vi "SeqMgr.Variables - Add, Replace.vi"(8 "error in (no error)":errorcluster, 9 "Name, Value":string[][](array[string]), 10 "Init":bool, 11 "SeqMgr in":refnum<class "SeqMgr.lvclass">) -> (0 "error out":errorcluster, 3 "SeqMgr out":refnum<class "SeqMgr.lvclass">)   [LabVIEW 2024, in "EQMF.lvlib" / "SeqMgr.lvlib" / "SeqMgr.lvclass"]
uses:
  SeqMgr.lvclass
  SeqMgr.lvclass/SeqMgr.ctl
  Strings/String Utils.lvlib
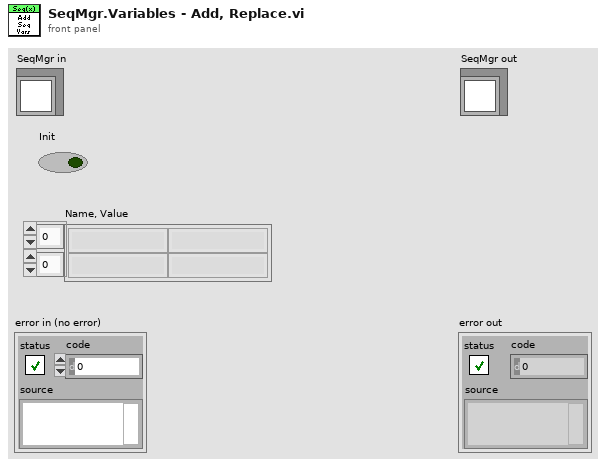
[diagram p1: front panel]
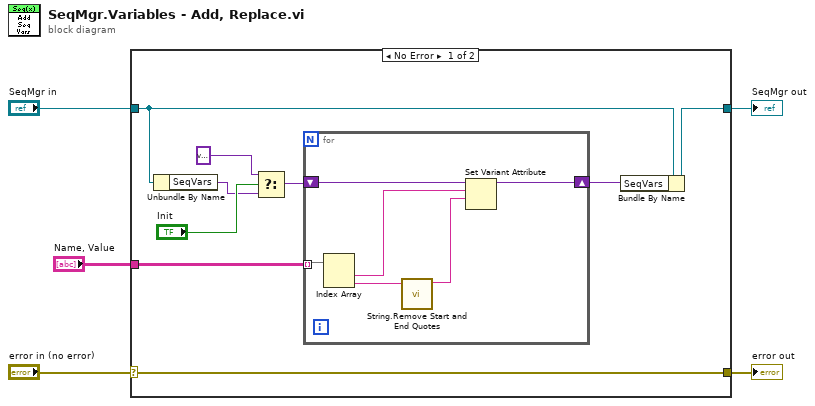
[diagram p0: block diagram]
diagram:
  n1 = case shown="No Error" "error in (no error)" {
    selector: "error in (no error)" -> [w14 w22]
    tunnel: [w14 w22] -> w4
    tunnel: [w13 w21] -> w2
    tunnel: "SeqMgr in" -> [w12 w21]
    tunnel: "Name, Value" -> [w10 _]
    frame No Error {
      n2 = Unbundle By Name(w12) -> ("SeqVars"=w8:variant)
      n3 = Select(t=variant, s="Init", f=w8) -> (s? t:f=w6:variant)
      n4 = for {
        shift-right: [w19] -> w11
        shift-left: w6 -> [w20]
        tunnel: w10 -> [w18] mode=indexing
        n5 = Index Array(array=w18) -> (element #1=w17:string, element #2=w16:string)  [unwired: 2 in]
        n6 = call "String.Remove Start and End Quotes.vi"("String In"=w16) -> ("String Out"=w15:string)  [unwired: 9 in, 1 out]
        n7 = Set Variant Attribute(Variant=w20, name=w17, value=w15) -> (Variant out=w19:variant)  [unwired: 1 in, 2 out]
      }
      n8 = Bundle By Name(cluster=w12, "SeqVars"=w11) -> (w13:refnum<class "SeqMgr.lvclass">)
    }
    frame Error {
    }
  }
  "error out" <- w4
  "SeqMgr out" <- w2
